vi "TableDisplay_init.vi"(8 "error in (no error)":errorcluster, 11 "AdvanceTable in":refnum<class "AdvanceTable.lvclass">) -> (0 "error out":errorcluster, 3 "AdvanceTable out":refnum<class "AdvanceTable.lvclass">)   [LabVIEW 2015, in "ActorManagement.lvlib" / "AdvanceTable.lvclass"]
uses:
  AdvanceTable.lvclass
  AdvanceTable.lvclass/AdvanceTable.ctl
  Scroll/Scroller.lvclass
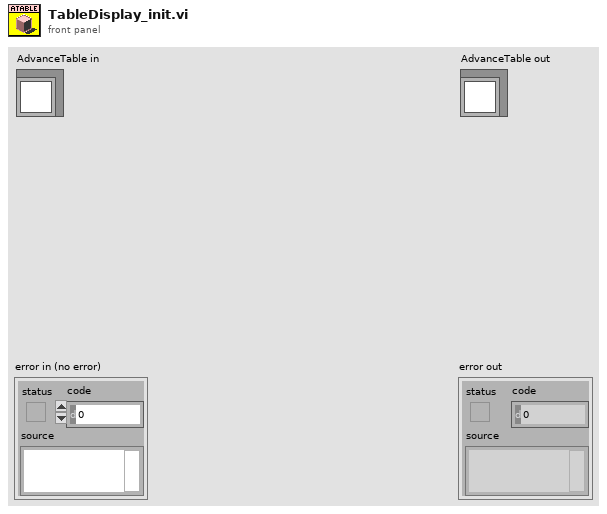
[diagram p1: front panel]
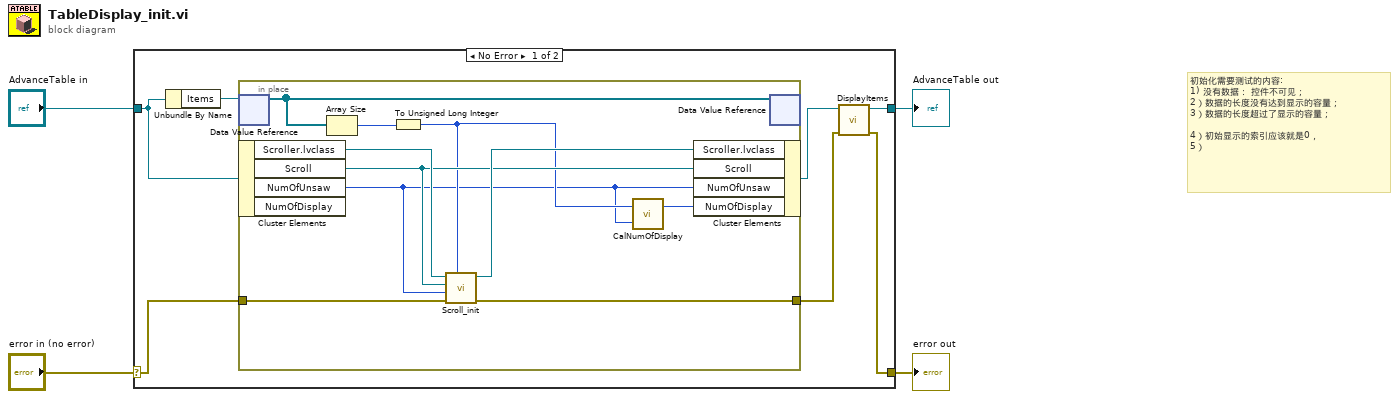
[diagram p0: block diagram]
diagram:
  # "初始化需要测试的内容:\n1) 没有数据： 控件不可见；\n2）数据的长度没有达到显示的容量；\n3）数据的长度超过了显示的容量；\n\n4）初始显示的索引应该就是0，\n5）"
  n1 = case shown="No Error" "error in (no error)" {
    selector: "error in (no error)" -> [w9 w23]
    tunnel: [w6 w23] -> w3
    tunnel: [w5 w22] -> w1
    tunnel: "AdvanceTable in" -> [w10 w22]
    frame No Error {
      n2 = Unbundle By Name(w10) -> ("Items"=w11:refnum<data-value>)
      n3 = in-place {
        in-place-border: w9 -> [w21]
        in-place-border: [w15] -> w7
        n4 = in-place-dvr #1(w11) -> (w18:refnum<class "TableItem.lvclass">[])  [unwired: 1 out]
        n5 = in-place-cluster #2(w10) -> ("Scroller.lvclass"=w20:refnum<class "Scroller.lvclass">, "Scroll"=w16:refnum<vi>, "NumOfUnsaw"=w13:u32)  [unwired: 1 out]
        n6 = Array Size(array=w18) -> (size(s)=w19:i32)
        n7 = To Unsigned Long Integer(number=w19) -> (unsigned 32bit integer=w14:u32)
        n8 = call "Scroll_init.vi"("Sum"=w14, "error in (no error)"=w21, "Index"=w13, "Scroll"=w16, "Scroller in"=w20) -> ("error out"=w15:errorcluster, "Scroller out"=w17:refnum<class "Scroller.lvclass">)  [unwired: 5 in]
        n9 = call "CalNumOfDisplay.vi"("IndexOfBase"=w13, "DataSum"=w14) -> ("NumOfDisplay"=w12:u32)  [unwired: 1 in]
        n10 = in-place-cluster #2("Scroller.lvclass"=w17, "Scroll"=w16, "NumOfUnsaw"=w13, "NumOfDisplay"=w12) -> (w8:refnum<class "AdvanceTable.lvclass">)
        n11 = in-place-dvr #1(w18) -> ()  [unwired: 2 out]
      }
      n12 = call "DisplayItems.vi"("error in (no error)"=w7, "AdvanceTable in"=w8) -> ("error out"=w6:errorcluster, "AdvanceTable out"=w5:refnum<class "AdvanceTable.lvclass">)  [unwired: 8 in]
    }
    frame Error {
    }
  }
  "error out" <- w3
  "AdvanceTable out" <- w1
